vi "geolocatorSettings.vi"() -> ()   [LabVIEW 2018]
panel:
  in  "Tab Control":enum32{"Page 1", "Page 2"}(tab)
  in  "String":string
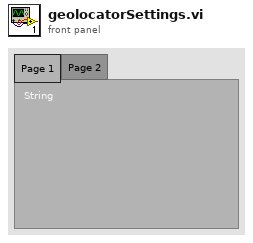
[diagram p1: front panel]
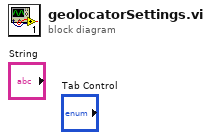
[diagram p0: block diagram]
diagram:
